vi "Write Required Digits of Precision.vi"(10 "Required Digits of Precision":u8=6, 11 "Floating Point in":refnum<class "Floating Point.lvclass">) -> (3 "Floating Point out":refnum<class "Floating Point.lvclass">)   [LabVIEW 2018, in "Floating Point.lvclass"]
uses:
  Floating Point.lvclass
  Floating Point.lvclass/Floating Point.ctl
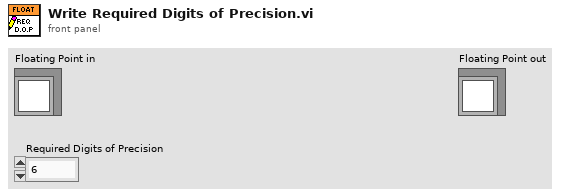
[diagram p1: front panel]
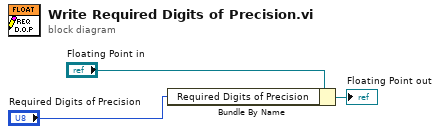
[diagram p0: block diagram]
diagram:
  n1 = Bundle By Name(cluster="Floating Point in", "Required Digits of Precision"="Required Digits of Precision") -> (→"Floating Point out":refnum<class "Floating Point.lvclass">)
